vi "List Nodes.vi"(8 "error in (no error)":errorcluster, 11 "Test Result in":refnum<class "Test Result.lvclass">) -> (0 "error out":errorcluster, 2 "Nodes":string[](array[string]), 3 "Test Result out":refnum<class "Test Result.lvclass">)   [LabVIEW 2013, in "Caraya.lvlib" / "Test Result.lvclass"]
uses:
  Test Result.lvclass
  Test Result.lvclass/Test Result.ctl
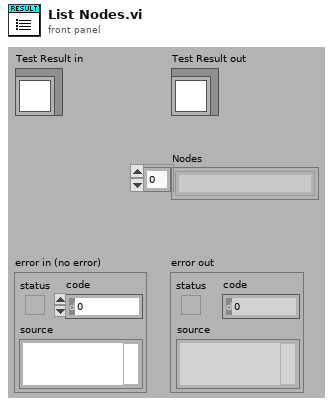
[diagram p1: front panel]
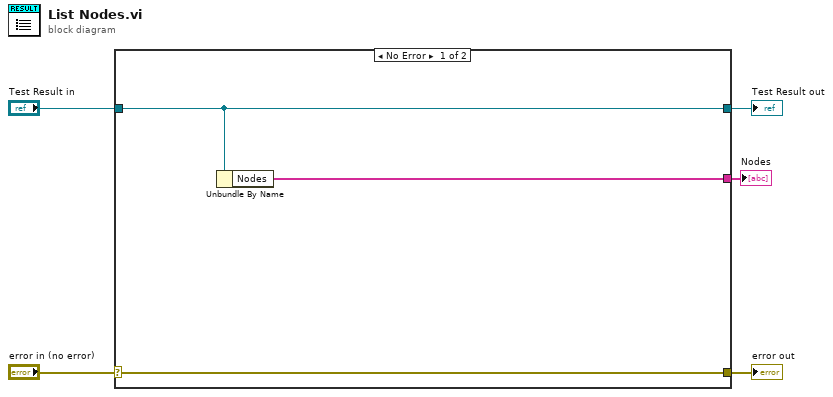
[diagram p0: block diagram]
diagram:
  n1 = case shown="No Error" "error in (no error)" {
    selector: "error in (no error)" -> [w7 w10]
    tunnel: [w7 w10] -> w4
    tunnel: [w8 w9] -> w2
    tunnel: "Test Result in" -> [w8 w9]
    tunnel: [w6 _] -> w1
    frame No Error {
      n2 = Unbundle By Name(w8) -> ("Nodes"=w6:string[])
    }
    frame Error {
    }
  }
  "error out" <- w4
  "Test Result out" <- w2
  "Nodes" <- w1
